vi "SweepCtrlPulseDeltaCurrent_ver2.0.vi"(4 "# of PLC":i16=10, 7 "Keithley 6221":T1={"Delta "=FALSE, "Const I "=FALSE, "Pulse Delta "=FALSE, "Sine Wave "=FALSE, "From I_HI (A)"=0.0, "From I (A)"=0.0, "I_LO (A)"=0.0, "From I_H (A)"=0.0, "I_L (A)"=0.0, "Freq (Hz)"=13.259, "From I_Sin (A)"=0.0, "DC Offset (A)"=0.0, "Delay Time (s)"=1.0, "Pulse Width (s)"=0.012, "Delay (s)"=0.011966, "To I (A)"=0.0, "ASymmetric?"=FALSE, "To I_HI (A)"=0.0, "To I_H (A)"=0.0, "To I_Sin (A)"=0.0, "GPIB ADR"=0, "Sweep Mode"=0, "Delta Unit"="V", "2182A range (V)"=0.01, "6221 Compliance (V)"=10.0} {"Sweep Mode" items=["Linear", "Log", "Exp", "Inverse", "Manual"]; "GPIB ADR" items=["None"=0, "12"=12, "13"=13]; "To I_Sin (A)" format="%#.5p"; "To I_H (A)" format="%#.5p"; "To I_HI (A)" format="%#.5p"; "To I (A)" format="%#.5p"; "Delay (s)" format="%.3p"; "Pulse Width (s)" format="%.3p"; "Delay Time (s)" format="%#.5p"; "DC Offset (A)" format="%#.5p"; "From I_Sin (A)" format="%#.5p"; "Freq (Hz)" format="%#_6p"; "I_L (A)" format="%#.5p"; "From I_H (A)" format="%#.5p"; "I_LO (A)" format="%#.5p"; "From I (A)" format="%#.5p"; "From I_HI (A)" format="%#.5p"}, 8 "error in (no error)":errorcluster, 9 "Set pt change flag":bool, 10 "DC St. Pt.":dbl, 11 "GPIB ADR":u16) -> (0 "error out":errorcluster)   [LabVIEW 2012]
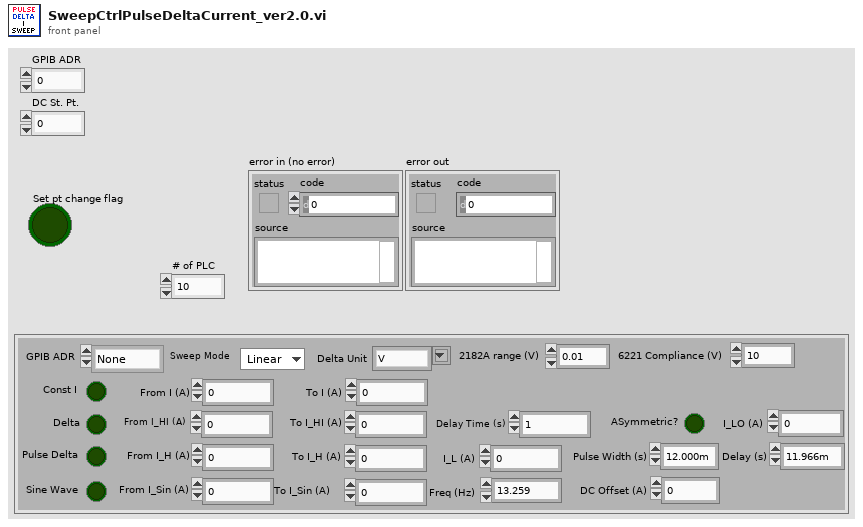
[diagram p1: front panel]
types:
  T1 = cluster{"Delta ":bool, "Const I ":bool, "Pulse Delta ":bool, "Sine Wave ":bool, "From I_HI (A)":dbl, "From I (A)":dbl, "I_LO (A)":dbl, "From I_H (A)":dbl, "I_L (A)":dbl, "Freq (Hz)":dbl, "From I_Sin (A)":dbl, "DC Offset (A)":dbl, "Delay Time (s)":dbl, "Pulse Width (s)":dbl, "Delay (s)":dbl, "To I (A)":dbl, "ASymmetric?":bool, "To I_HI (A)":dbl, "To I_H (A)":dbl, "To I_Sin (A)":dbl, "GPIB ADR":u16, "Sweep Mode":u8, "Delta Unit":string, "2182A range (V)":dbl, "6221 Compliance (V)":dbl}
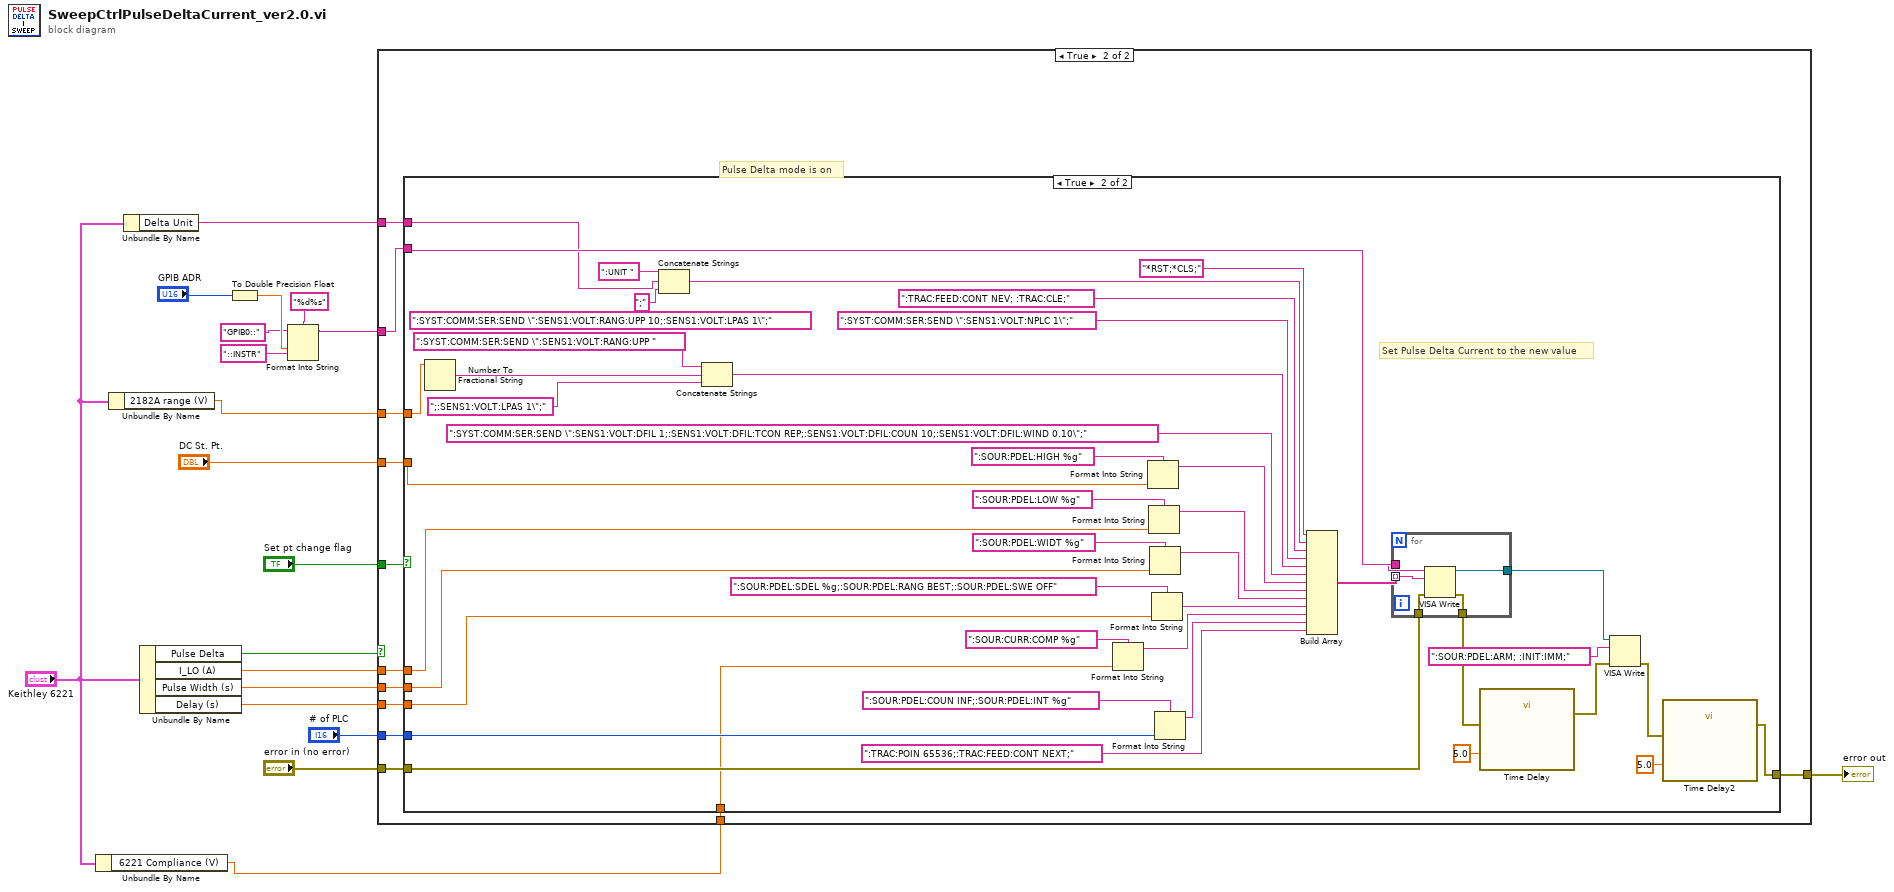
[diagram p0: block diagram]
diagram:
  n1 = Unbundle By Name("Keithley 6221") -> ("6221 Compliance (V)"=w1:dbl)
  n2 = Unbundle By Name("Keithley 6221") -> ("2182A range (V)"=w2:dbl)
  n3 = Unbundle By Name("Keithley 6221") -> ("Delta Unit"=w3:string)
  n4 = Unbundle By Name("Keithley 6221") -> ("Pulse Delta"=w14:bool, "I_LO (A)"=w11:dbl, "Pulse Width (s)"=w10:dbl, "Delay (s)"=w6:dbl)
  n5 = To Double Precision Float(number="GPIB ADR") -> (double precision float=w18:dbl)
  n6 = Format Into String(format string="%d%s" ("Removes all labels from the string"), initial string="GPIB0::", w18, "::INSTR") -> (resulting string=w13:string)  [unwired: 1 in, 1 out]
  n7 = case shown="True" w14 {
    tunnel: "Set pt change flag" -> [_ w32]
    tunnel: w13 -> [_ w31]
    tunnel: "DC St. Pt." -> [_ w30]
    tunnel: w11 -> [_ w29]
    tunnel: w10 -> [_ w28]
    tunnel: "error in (no error)" -> [w20 w27]
    tunnel: [w20 w26] -> w8
    tunnel: w6 -> [_ w25]
    tunnel: "# of PLC" -> [_ w24]
    tunnel: w2 -> [_ w23]
    tunnel: w1 -> [_ w22]
    tunnel: w3 -> [_ w21]
    frame False {
      # "Pulse Delta mode is off"
    }
    frame True {
      # "Pulse Delta mode is on"
      n8 = case shown="True" w32 {
        tunnel: w31 -> [_ w74]
        tunnel: w30 -> [_ w70]
        tunnel: w29 -> [_ w65]
        tunnel: w28 -> [_ w57]
        tunnel: w27 -> [w33 w66]
        tunnel: [w33 w45] -> w26
        tunnel: w25 -> [_ w59]
        tunnel: w24 -> [_ w54]
        tunnel: w23 -> [_ w39]
        tunnel: w22 -> [_ w41]
        tunnel: w21 -> [_ w34]
        frame False {
          # "Set Values are not changed"
        }
        frame True {
          (unwired) ":SYST:COMM:SER:SEND \":SENS1:VOLT:RANG:UPP 10;:SENS1:VOLT:LPAS 1\";" ("format string")
          # "Set Pulse Delta Current to the new value"
          n9 = Number To Fractional String(number=w39) -> (F-format string=w37:string)  [unwired: 3 in]
          n10 = Concatenate Strings(":UNIT " ("write buffer"), w34, ";" ("string")) -> (w72:string)
          n11 = Concatenate Strings(":SYST:COMM:SER:SEND \":SENS1:VOLT:RANG:UPP " ("format string"), w37, ";:SENS1:VOLT:LPAS 1\";" ("format string")) -> (w35:string)
          n12 = Format Into String(format string=":SOUR:CURR:COMP %g", w41) -> (resulting string=w40:string)  [unwired: 2 in, 1 out]
          n13 = Format Into String(format string=":SOUR:PDEL:HIGH %g", w70) -> (resulting string=w71:string)  [unwired: 2 in, 1 out]
          n14 = Format Into String(format string=":SOUR:PDEL:LOW %g", w65) -> (resulting string=w69:string)  [unwired: 2 in, 1 out]
          n15 = Format Into String(format string=":SOUR:PDEL:WIDT %g", w57) -> (resulting string=w51:string)  [unwired: 2 in, 1 out]
          n16 = Format Into String(format string=":SOUR:PDEL:SDEL %g;:SOUR:PDEL:RANG BEST;:SOUR:PDEL:SWE OFF", w59) -> (resulting string=w68:string)  [unwired: 2 in, 1 out]
          n17 = Format Into String(format string=":SOUR:PDEL:COUN INF;:SOUR:PDEL:INT %g", w54) -> (resulting string=w50:string)  [unwired: 2 in, 1 out]
          n18 = Build Array("*RST;*CLS;" ("write buffer"), w72, ":TRAC:FEED:CONT NEV; :TRAC:CLE;" ("format string"), ":SYST:COMM:SER:SEND \":SENS1:VOLT:NPLC 1\";", w35, ":SYST:COMM:SER:SEND \":SENS1:VOLT:DFIL 1;:SENS1:VOLT:DFIL:TCON REP;:SENS1:VOLT:DFIL:COUN 10;:SENS1:VOLT:DFIL:WIND 0.10\";", w71, w69, w51, w68, w40, w50, ":TRAC:POIN 65536;:TRAC:FEED:CONT NEXT;" ("format string")) -> (w67:string[])
          n19 = for {
            tunnel: w67 -> [w81] mode=indexing
            tunnel: w74 -> [w80]
            tunnel: w66 -> [w79]
            tunnel: [w78] -> w46
            tunnel: [w77] -> w49
            n20 = VISA Write(VISA resource name=w80, write buffer=w81, error in (no error)=w79) -> (VISA resource name out=w78:refnum<visa-resource-name>, error out=w77:errorcluster)  [unwired: 1 out]
          }
          n21 = call "Time Delay"("error in (no error)"=w49, "Delay Time (s)"=5.0) -> ("error out"=w48:errorcluster)  [unwired: 9 in]
          n22 = VISA Write(VISA resource name=w46, write buffer=":SOUR:PDEL:ARM; :INIT:IMM;" ("format string"), error in (no error)=w48) -> (error out=w44:errorcluster)  [unwired: 2 out]
          n23 = call "Time Delay2"("error in (no error)"=w44, "Delay Time (s)"=5.0) -> ("error out"=w45:errorcluster)  [unwired: 9 in]
        }
      }
    }
  }
  "error out" <- w8
